vi "User32dllAPI.GetWindowTextLength.vi"(8 "error in (no error)":errorcluster, 11 "hWnd":i32) -> (0 "error out":errorcluster, 2 "length":i32, 3 "hWnd out":i32)   [LabVIEW 2019, in "Tools.lvlib"]
uses:
  Tools.lvlib
  user32.dll
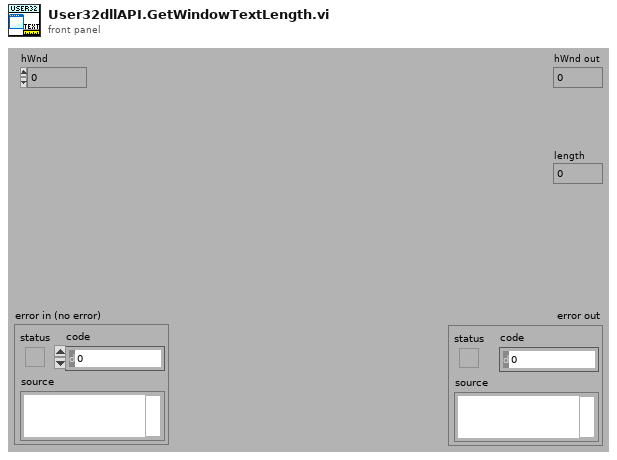
[diagram p1: front panel]
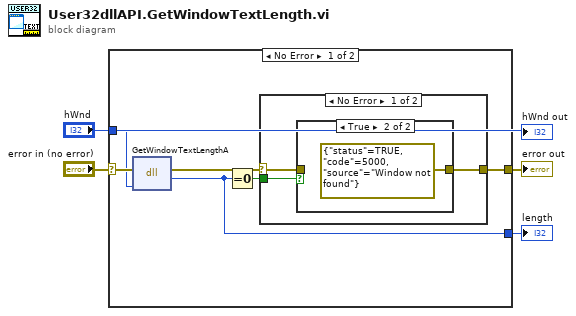
[diagram p0: block diagram]
diagram:
  n1 = case shown="No Error" "error in (no error)" {
    selector: "error in (no error)" -> [w9 w17]
    tunnel: [w7 w17] -> w3
    tunnel: "hWnd" -> [w6 _]
    tunnel: [w5 _] -> w2
    frame No Error {
      n2 = dll-call lib="USER32.DLL" fn="GetWindowTextLengthA"(error in=w9, "hwnd"=w6) -> (error out=w8:errorcluster, "length"=w5:i32)  [unwired: 3 in, 1 out]
      n3 = Equal To 0?(x=w5) -> (x = 0?=w10:bool)
      n4 = case shown="No Error" w8 {
        selector: w8 -> [w11 w16]
        tunnel: w10 -> [w13 _]
        tunnel: [w12 w16] -> w7
        frame No Error {
          n5 = case shown="True" w13 {
            tunnel: [w14 errorcluster {"status"=TRUE, "code"=5000, "source"="Window not found"} ("error out")] -> w12
            tunnel: w11 -> [w14 _]
            frame False {
            }
            frame True {
            }
          }
        }
        frame Error {
        }
      }
    }
    frame Error {
    }
  }
  "error out" <- w3
  "length" <- w2
  "hWnd out" <- "hWnd"
